vi "OCR_Get Text from bit lines.vi"(8 "Error":errorcluster, 11 "Bit Line Array":T1[](array[typedef])) -> (0 "Error Out":errorcluster, 3 "Text Out":T3[](array[typedef]), 4 "Status Of Each Line Out":bool[](array[boolean]))   [LabVIEW 2009]
doc: "Builds an array of strings from a bit line array."
uses:
  Controls/String_Picture/STRING_Line Display.ctl
  Controls/Cluster/Cluster_Bit array and line status.ctl
  Controls/String_Picture/String Char Normal.ctl
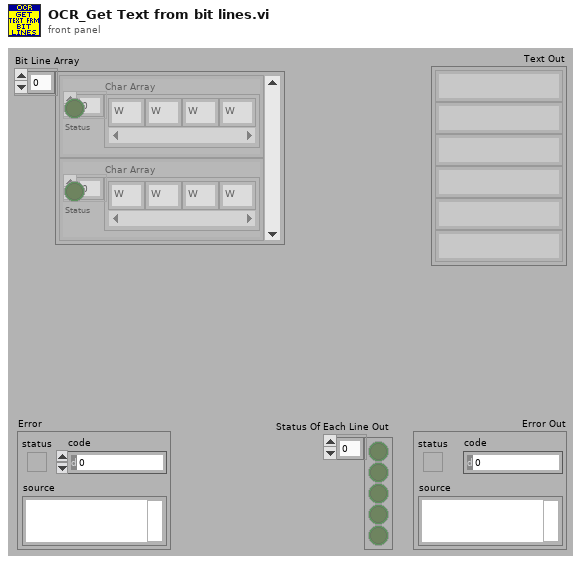
[diagram p1: front panel]
types:
  T1 = typedef "Cluster_Bit array and line status.ctl" = cluster{"Char Array":T2[], "Status":bool}
  T2 = typedef "String Char Normal.ctl" = string
  T3 = typedef "STRING_Line Display.ctl" = string
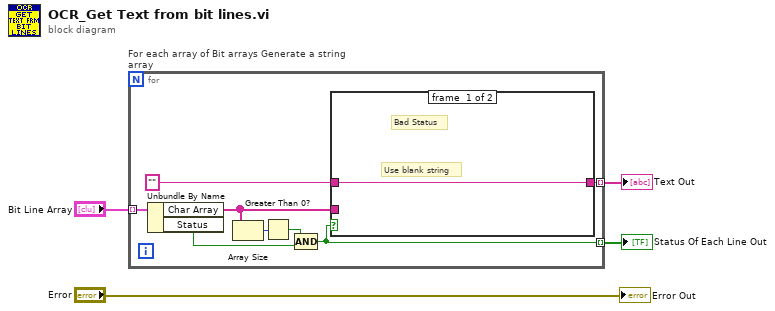
[diagram p0: block diagram]
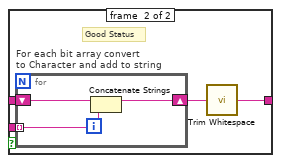
[diagram p2: hidden frame]
diagram:
  n1 = for "For each array of Bit arrays Generate a string array" {
    tunnel: "Bit Line Array" -> [w12] mode=indexing
    tunnel: [w11] -> w2 mode=indexing
    tunnel: [w5] -> w3 mode=indexing
    n2 = Unbundle By Name(w12) -> ("Char Array"=w9:T2[], "Status"=w7:bool)
    n3 = Array Size(array=w9) -> (size(s)=w8:i32)
    n4 = Greater Than 0?(x=w8) -> (x > 0?=w6:bool)
    n5 = Compound Arithmetic op=AND(w6, w7) -> (w5:bool)
    n6 = case shown="True" w5 {
      tunnel: w9 -> [_ w17]
      tunnel: [w13 w14] -> w11
      tunnel: "" -> [w13 w16]
      frame #0 {
        # "Use blank string"
        # "Bad Status"
      }
      frame #1 {
        # "Good Status"
        n7 = for "For each bit array convert\nto Character and add to string" {
          tunnel: w17 -> [w18] mode=indexing
          shift-right: [w20] -> w15
          shift-left: w16 -> [w19]
          n8 = Concatenate Strings(w19, w18) -> (w20:string)
        }
        n9 = call <vilib>:"Trim Whitespace.vi"("string"=w15) -> ("trimmed string"=w14:string)  [unwired: 1 in]
      }
    }
  }
  "Text Out" <- w2
  "Status Of Each Line Out" <- w3
  "Error Out" <- "Error"
